vi "Write Temp Data HDF5 File.vi"(8 "Error In":errorcluster, 10 "Photon Time Stamps":i64[](array[numeric]), 11 "Photon Detector IDs":u8[](array[numeric])) -> (0 "Error Out":errorcluster, 3 "HDF5 File Path":path)   [LabVIEW 2010]
uses:
  <vilib>/addons/h5labview2/file/H5Fmode.ctl
  <vilib>/addons/h5labview2/dataset/H5Dwrite.llb/H5Dwrite.xnode
  <vilib>/addons/h5labview2/base/lib_path.vi
  <vilib>/addons/h5labview2/base/H5Equery.vi
  <vilib>/addons/h5labview2/file/H5F.lvlib
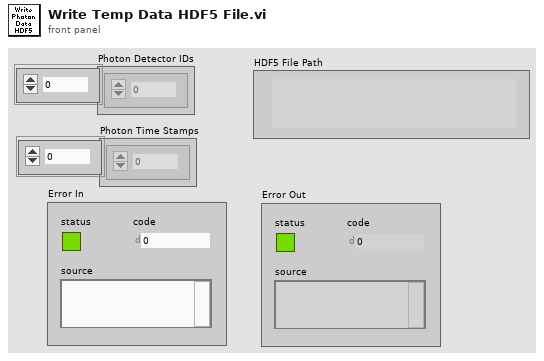
[diagram p1: front panel]
types:
  T1 = typedef "H5F.lvlib/H5Fmode.ctl" = enum16{"read-only", "read-write", "overwrite", "create new", "open or create"}
  T2 = typedef "hid_t.ctl" = i32
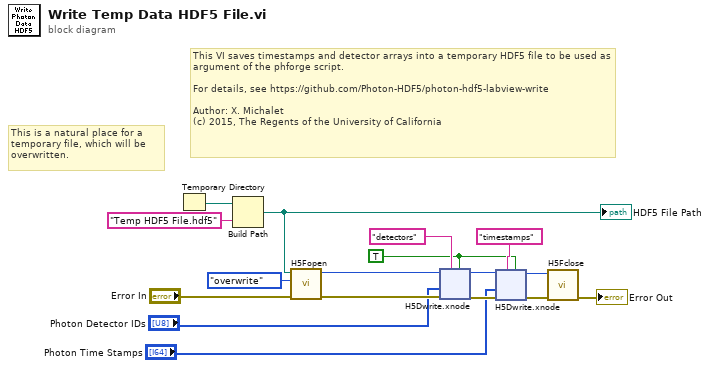
[diagram p0: block diagram]
diagram:
  w6 = TRUE ("replace? (F)")
  # "This is a natural place for a temporary file, which will be overwritten."
  # "This VI saves timestamps and detector arrays into a temporary HDF5 file to be used as argument of the phforge script.\n\nFor details, see https://github.com/Photon-HDF5/photon-hdf5-labview-write\n\nAuthor: X. Michalet\n(c) 2015, The Regents of the University of California"
  n1 = Temporary Directory() -> (w16:path)
  n2 = Build Path(base path=w16, name or relative path="Temp HDF5 File.hdf5") -> (appended path=w14:path)
  "HDF5 File Path" <- w14
  n3 = call <vilib>:"H5Fopen.vi"("error in (no error)"="Error In", "mode (read-only)"=H5Fmode."overwrite", "path"=w14) -> ("error out"=w12:errorcluster, "ref out"=w11:T2)  [unwired: 7 in]
  n4 = xnode "H5Dwrite.xnode"("replace? (F)"=w6, "dataset name"="detectors" ("name"), "error in (no error)"=w12, "data"="Photon Detector IDs", "ref in"=w11) -> ("error out"=w8:errorcluster, "ref out"=w9:i32)  [unwired: 2 in, 1 out]
  n5 = xnode "H5Dwrite.xnode"("replace? (F)"=w6, "dataset name"="timestamps", "error in (no error)"=w8, "data"="Photon Time Stamps", "ref in"=w9) -> ("error out"=w5:errorcluster, "ref out"=w4:i32)  [unwired: 2 in, 1 out]
  n6 = call <vilib>:"H5Fclose.vi"("error in (no error)"=w5, "ref"=w4) -> ("error out"=→"Error Out":errorcluster)  [unwired: 9 in]
